vi "read write.vi"() -> ()   [LabVIEW 2011]
panel:
  in  "Tab Control":T1(tab)
  out "Read Text":string
  in  "Write Text":string="This text will be\nwritten to file."
  in  "Path":path=path "C:/write-read example.txt"
  in  "Path 2":path
  out "Read Text 2":string
  in  "Write Text 2":string="This text will be\nwritten to file."
  in  "Path 3":path
  in  "Write Text 3":string="This text will be\\n\nwritten to file.\\n\\r"
  out "Read Text 3":string
  in  "Path 4":path
  out "Read Text 4":string
  in  "Write Text 4":string="This text will be\nwritten to file."
  in  "Path 5":path
  in  "Count":i32=-1
  out "Read Text Array":string[](array[string])
  in  "Write Text 5":string="This text will be\nwritten to file."
  # "Both the Write and Read Text File functions \ncan identify files using a path.  This case shows \nhow the functions will execute when a path is defined."
  # "The Write and Read Text File functions can also \nidentify files using the file refnum, provided by \nthe Open/Create/Replace function."
  # "By default, LabVIEW Converts the EOL characters \ndepending on the platform.  In this case the EOL \nConvert option has been disabled on the Write and \nRead Text File by right-clicking on the function and \nunchecking that option.  Notice that the text file \nthat is created does not have the proper formatting."
  # "The Read Lines option will allow the Read Text File function \nto read lines instead of characters.  In this case the Read \nLines function has been enabled by right-clicking the Read \nText File function and checking that option.  Notice that \nonly one line is read by default."
  # "This case also enables the Read Lines option, but uses \nthe Count input to the Read Text File function, which \ndefines the number of lines to read.  This causes the \noutput of the function to be an array of strings, each \nelement corresponding to a line.  The Count parameter \ncan be set to -1 to read the entire file."
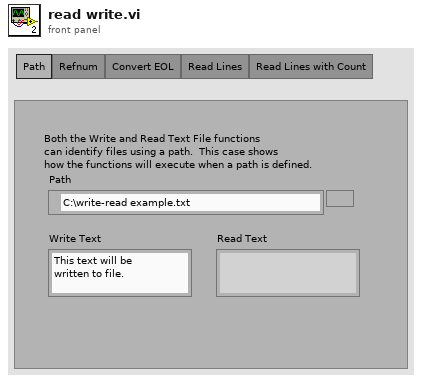
[diagram p1: front panel]
types:
  T1 = enum32{"Path", "Refnum", "Convert EOL", "Read Lines", "Read Lines with Count"}
  T2 = enum16{"open", "replace", "create", "open or create", "replace or create", "replace or create with confirmation"}
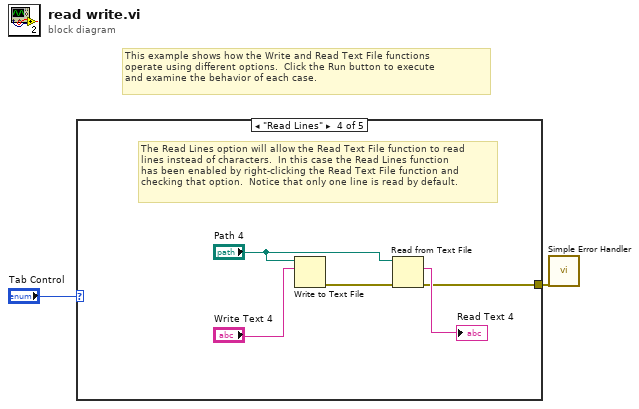
[diagram p0: block diagram]
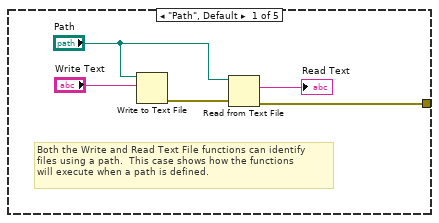
[diagram p2: hidden frame]
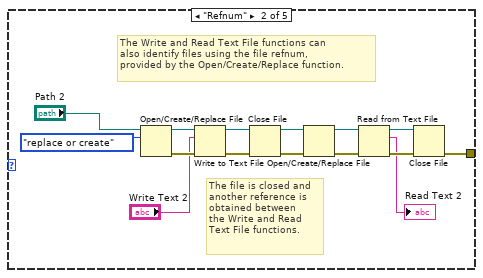
[diagram p3: hidden frame]
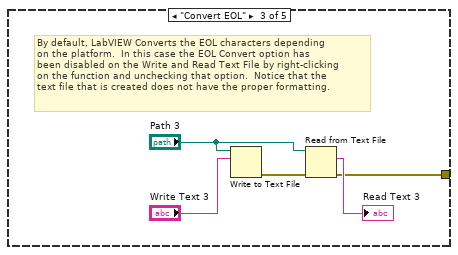
[diagram p4: hidden frame]
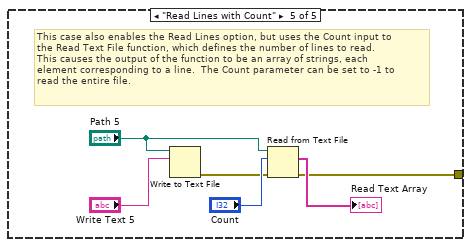
[diagram p5: hidden frame]
diagram:
  # "This example shows how the Write and Read Text File functions \noperate using different options.  Click the Run button to execute \nand examine the behavior of each case."
  n1 = case shown="\"Read Lines\"" "Tab Control" {
    tunnel: [w4 w17 w24 w29 w34] -> w1
    frame "Path", Default {
      # "Both the Write and Read Text File functions can identify \nfiles using a path.  This case shows how the functions \nwill execute when a path is defined."
      n2 = Write to Text File(file (use dialog)="Path", text="Write Text") -> (error out=w6:errorcluster)  [unwired: 2 in, 2 out]
      n3 = Read from Text File(file (use dialog)="Path", error in=w6) -> (text=→"Read Text":string, error out=w4:errorcluster)  [unwired: 2 in, 2 out]
    }
    frame "Refnum" {
      # "The Write and Read Text File functions can \nalso identify files using the file refnum, \nprovided by the Open/Create/Replace function."
      # "The file is closed and \nanother reference is \nobtained between \nthe Write and Read \nText File functions."
      n4 = Open/Create/Replace File(file path (use dialog)="Path 2", operation (0:open)=T2."replace or create") -> (refnum out=w20:refnum<file>, error out=w22:errorcluster)  [unwired: 4 in, 1 out]
      n5 = Write to Text File(file (use dialog)=w20, text="Write Text 2", error in=w22) -> (refnum out=w14:refnum<file>, error out=w10:errorcluster)  [unwired: 1 in, 1 out]
      n6 = Close File(refnum=w14, error in=w10) -> (path=w13:path, error out=w12:errorcluster)
      n7 = Open/Create/Replace File(file path (use dialog)=w13, error in=w12) -> (refnum out=w11:refnum<file>, error out=w9:errorcluster)  [unwired: 4 in, 1 out]
      n8 = Read from Text File(file (use dialog)=w11, error in=w9) -> (refnum out=w19:refnum<file>, text=→"Read Text 2":string, error out=w18:errorcluster)  [unwired: 2 in, 1 out]
      n9 = Close File(refnum=w19, error in=w18) -> (error out=w17:errorcluster)  [unwired: 1 out]
    }
    frame "Convert EOL" {
      # "By default, LabVIEW Converts the EOL characters depending \non the platform.  In this case the EOL Convert option has \nbeen disabled on the Write and Read Text File by right-clicking \non the function and unchecking that option.  Notice that the \ntext file that is created does not have the proper formatting."
      n10 = Write to Text File(file (use dialog)="Path 3", text="Write Text 3") -> (error out=w25:errorcluster)  [unwired: 2 in, 2 out]
      n11 = Read from Text File(file (use dialog)="Path 3", error in=w25) -> (text=→"Read Text 3":string, error out=w24:errorcluster)  [unwired: 2 in, 2 out]
    }
    frame "Read Lines" {
      # "The Read Lines option will allow the Read Text File function to read \nlines instead of characters.  In this case the Read Lines function \nhas been enabled by right-clicking the Read Text File function and \nchecking that option.  Notice that only one line is read by default."
      n12 = Write to Text File(file (use dialog)="Path 4", text="Write Text 4") -> (error out=w30:errorcluster)  [unwired: 2 in, 2 out]
      n13 = Read from Text File(file (use dialog)="Path 4", error in=w30) -> (text=→"Read Text 4":string, error out=w29:errorcluster)  [unwired: 2 in, 2 out]
    }
    frame "Read Lines with Count" {
      # "This case also enables the Read Lines option, but uses the Count input to \nthe Read Text File function, which defines the number of lines to read.  \nThis causes the output of the function to be an array of strings, each \nelement corresponding to a line.  The Count parameter can be set to -1 to \nread the entire file."
      n14 = Write to Text File(file (use dialog)="Path 5", text="Write Text 5") -> (error out=w35:errorcluster)  [unwired: 2 in, 2 out]
      n15 = Read from Text File(file (use dialog)="Path 5", count="Count", error in=w35) -> (text=→"Read Text Array":string[], error out=w34:errorcluster)  [unwired: 1 in, 2 out]
    }
  }
  n16 = call <vilib>:"Simple Error Handler.vi"("error in (no error)"=w1) -> ()  [unwired: 4 in, 5 out]
